vi "CreateGraphFromName.vi"(2 "GraphTypeToCreate":string, 5 "error in (no error)":errorcluster) -> (14 "GraphCreated":refnum<class "Graph.lvclass">, 19 "error out":errorcluster)   [LabVIEW 2016, in "Graph.lvclass"]
uses:
  <resource>/Framework/Providers/Open_GDS/UML/Graph_class/Graph.lvclass
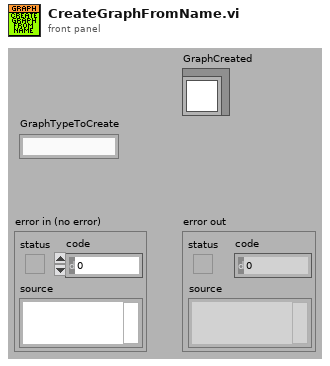
[diagram p1: front panel]
types:
  T1 = typedef "Graph.lvclass/ClassAttributes.ctl" = cluster{"NODE_PROT":refnum<class "AbstractNode.lvclass">[], "NodeNames":string[], "EDGE_PROT":refnum<class "AbstractEdge.lvclass">[], "EdgeNames":string[], "GraphTypes":refnum<class "Graph.lvclass">[], "GraphTypeNames":string[], "NodeTypes":refnum<class "AbstractNode.lvclass">[], "EdgeTypes":refnum<class "AbstractEdge.lvclass">[], "NodeTypeNames":string[], "EdgeTypeNames":string[]}
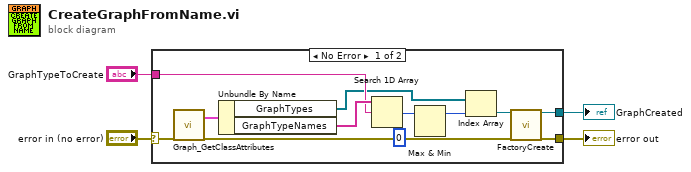
[diagram p0: block diagram]
diagram:
  n1 = case shown="No Error" "error in (no error)" {
    selector: "error in (no error)" -> [w16 w17]
    tunnel: [w9 w17] -> w3
    tunnel: [w8 _] -> w2
    tunnel: "GraphTypeToCreate" -> [w13 _]
    frame No Error {
      n2 = call <resource>:"Graph_GetClassAttributes.vi"("error in (no error)"=w16) -> ("Class attribute"=w15:T1, "error out"=w10:errorcluster)  [unwired: 15 in, 2 out]
      n3 = Unbundle By Name(w15) -> ("GraphTypes"=w12:refnum<class "Graph.lvclass">[], "GraphTypeNames"=w14:string[])
      n4 = Search 1D Array(1D array=w14, element=w13) -> (index of element=w7:i32)  [unwired: 1 in]
      n5 = Max & Min(x=w7, y=0) -> (max(x,y)=w6:i32)  [unwired: 1 out]
      n6 = Index Array(array=w12, index=w6) -> (element=w11:refnum<class "Graph.lvclass">)
      n7 = call-dynamic "FactoryCreate.vi"("reference in"=w11, "error in (no error)"=w10) -> ("reference out"=w8:refnum<class "Graph.lvclass">, "error out"=w9:errorcluster)  [unwired: 16 in]
    }
    frame Error {
    }
  }
  "error out" <- w3
  "GraphCreated" <- w2
